vi "ExSubSwitchXnYCreateFileDisplay.vi"(2 "error in (no error)":errorcluster, 3 "File and Display Name":string, 4 "Pulser Handle":u32, 5 "Camera Handle":u32) -> (0 "error out":errorcluster, 1 "Handles Out":T1)   [LabVIEW 2010]
panel:
  # "ExSubCreateFileDisplay:\nThis is a SubVI that creates a file, display \nand image objects and returns the handles \nbundled in a cluster that includes a pulser \nand camera handle"
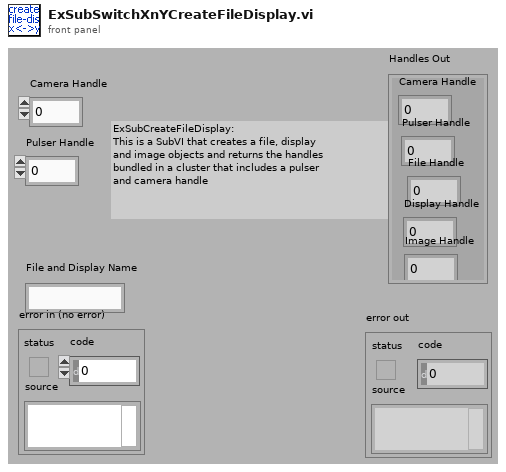
[diagram p1: front panel]
types:
  T1 = cluster{"Camera Handle":u32, "Pulser Handle":u32, "File Handle":u32, "Display Handle":u32, "Image Handle":u32}
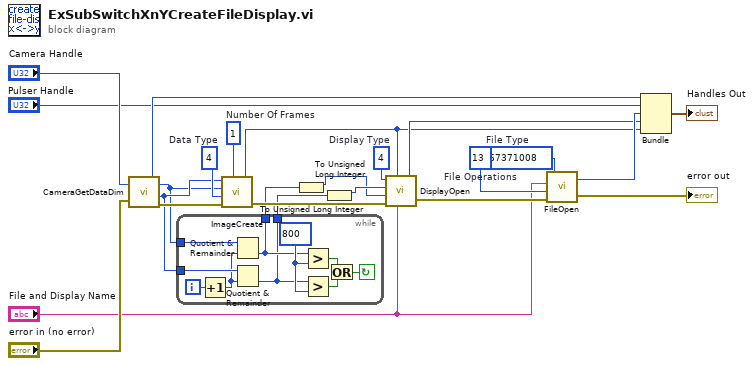
[diagram p0: block diagram]
diagram:
  w7 = u32 1  # Number Of Frames
  w8 = u32 4  # Display Type
  w9 = u32 4  # Data Type
  w11 = 13  # File Operations
  w12 = 67371008  # File Type
  n1 = call <userlib>:"CameraGetDataDim.vi"("Camera Handle"="Camera Handle", "error in"="error in (no error)") -> ("Camera Handle"=w18:u32, "Xdim"=w1:u32, "Ydim"=w2:u32, "error out"=w24:errorcluster)
  n2 = while {
    tunnel: w1 -> [w33]
    tunnel: w2 -> [w32]
    tunnel: [w27] -> w6
    tunnel: [w26] -> w5
    i -> [w31]
    stop <- w28 continue-if-true
    w34 = 800
    n3 = Increment(x=w31) -> (x+1=w25:i32)
    n4 = Quotient & Remainder(x=w33, y=w25) -> (floor(x/y)=w27:u32)  [unwired: 1 out]
    n5 = Quotient & Remainder(x=w32, y=w25) -> (floor(x/y)=w26:u32)  [unwired: 1 out]
    n6 = Greater?(x=w27, y=w34) -> (0:w30:bool)
    n7 = Greater?(x=w26, y=w34) -> (0:w29:bool)
    n8 = Or(x=w30, y=w29) -> (x .or. y?=w28:bool)
  }
  n9 = call <userlib>:"ImageCreate.vi"("X dimension"=w2, "Y dimension"=w1, "Data Type"=w9, "error in"=w24, "Number Of Frames"=w7) -> ("Image Handle"=w14:u32, "error out"=w23:errorcluster)
  n10 = To Unsigned Long Integer(number=w6) -> (unsigned 32bit integer=w3:u32)
  n11 = To Unsigned Long Integer(number=w5) -> (unsigned 32bit integer=w4:u32)
  n12 = call <userlib>:"DisplayOpen.vi"("Display Title"="File and Display Name", "Image Handle"=w14, "error in"=w23, "Display Height"=w3, "Display Width"=w4, "Display Type"=w8) -> ("error out"=w22:errorcluster, "Display Handle"=w15:u32)
  n13 = call <userlib>:"FileOpen.vi"("error in"=w22, "File Operations"=w11, "FileName"="File and Display Name", "File Type"=w12) -> ("error out"=→"error out":errorcluster, "File Handle"=w16:u32)
  n14 = Bundle("Camera Handle"=w18, "Pulser Handle"="Pulser Handle", "File Handle"=w16, "Display Handle"=w15, "Image Handle"=w14) -> (→"Handles Out":T1)  [unwired: 1 in]
